vi "Increment Reported Error.vi"(4 "Newly Reported Error":T1, 5 "Module Data in":T3) -> (0 "Index of the newly reported error in the OSI data structure":i32, 1 "No. of times the error was handled in the last second":u32, 2 "Module Data out (OSI data updated)":T3)   [LabVIEW 2023, in "Error Manager.lvlib"]
doc: "Blank VI with error handling."
uses:
  Error Manager.lvlib
  Module Data (cluster).ctl
  Handled Error (cluster).ctl
  Read-Unread Status (enum).ctl
  Display Order (enum).ctl
  Error in current one-second interval (cluster).ctl
  Reported Error (cluster).ctl
  Public API VIs/Pop-up New Error Dialogue Instruction (enum).ctl
panel:
  # "Input\nInputs to the VI"
  # "Development\nControls or indicators that are useful for development or testing, but which are not outputs of the VI."
  # "Output\nOutputs of the VI"
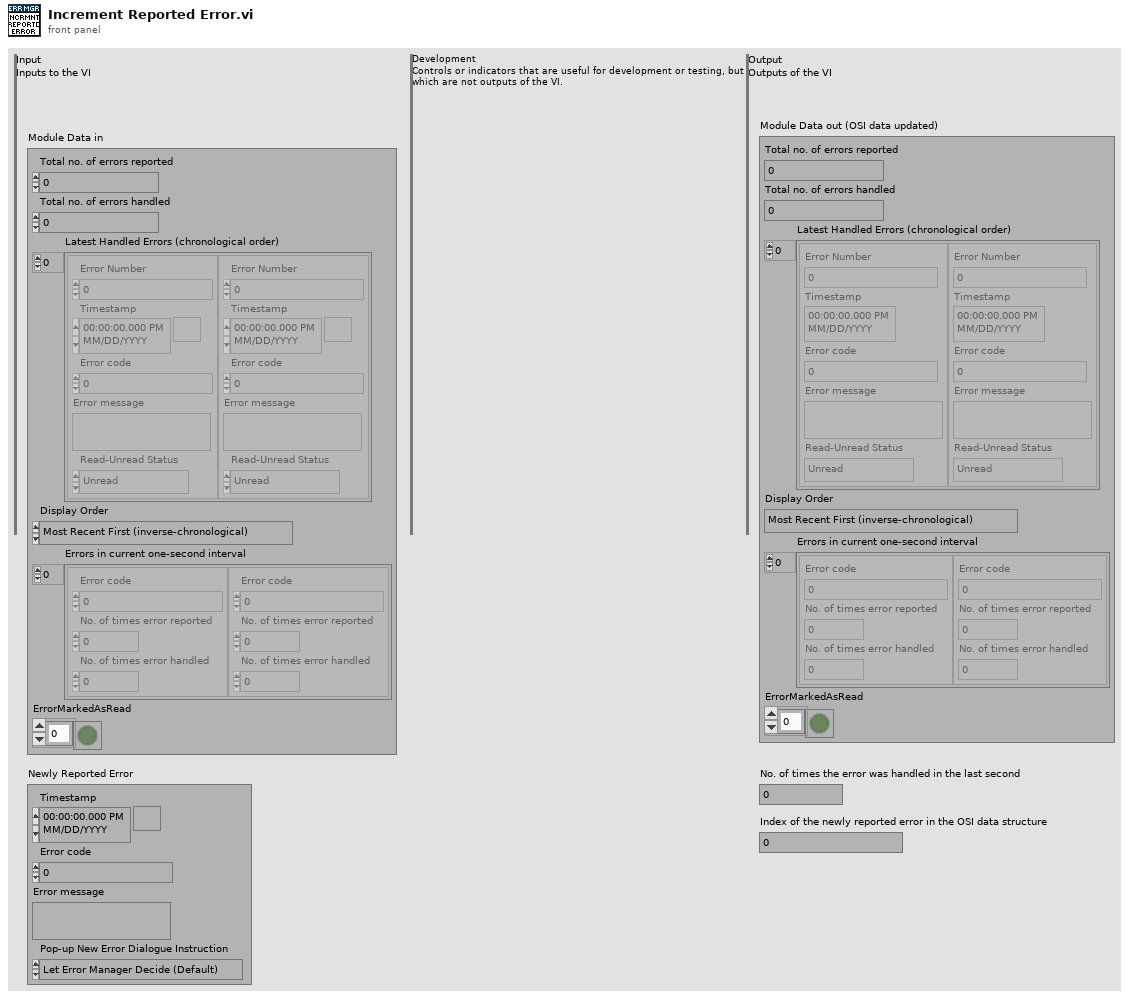
[diagram p1: front panel]
types:
  T1 = typedef "Error Manager.lvlib/Reported Error (cluster).ctl" = cluster{"Timestamp":timestamp, "Error code":i32, "Error message":string, "Pop-up New Error Dialogue Instruction":T2}
  T2 = typedef "Error Manager.lvlib/Pop-up New Error Dialogue Instruction (enum).ctl" = enum16{"Let Error Manager Decide (Default)", "Don't pop-up", "Pop-up"}
  T3 = typedef "Error Manager.lvlib/Module Data (cluster).ctl" = cluster{"Total no. of errors reported":i32, "Total no. of errors handled":i32, "Latest Handled Errors (chronological order)":T4[], "Display Order":T6, "Errors in current one-second interval":T7[], "ErrorMarkedAsRead":bool[]}
  T4 = typedef "Error Manager.lvlib/Handled Error (cluster).ctl" = cluster{"Error Number":i32, "Timestamp":timestamp, "Error code":i32, "Error message":string, "Read-Unread Status":T5}
  T5 = typedef "Error Manager.lvlib/Read-Unread Status (enum).ctl" = enum16{"Unread", "Read"}
  T6 = typedef "Error Manager.lvlib/Display Order (enum).ctl" = enum16{"Most Recent First (inverse-chronological)", "Oldest First (chronological)"}
  T7 = typedef "Error Manager.lvlib/Error in current one-second interval (cluster).ctl" = cluster{"Error code":i32, "No. of times error reported":u32, "No. of times error handled":u32}
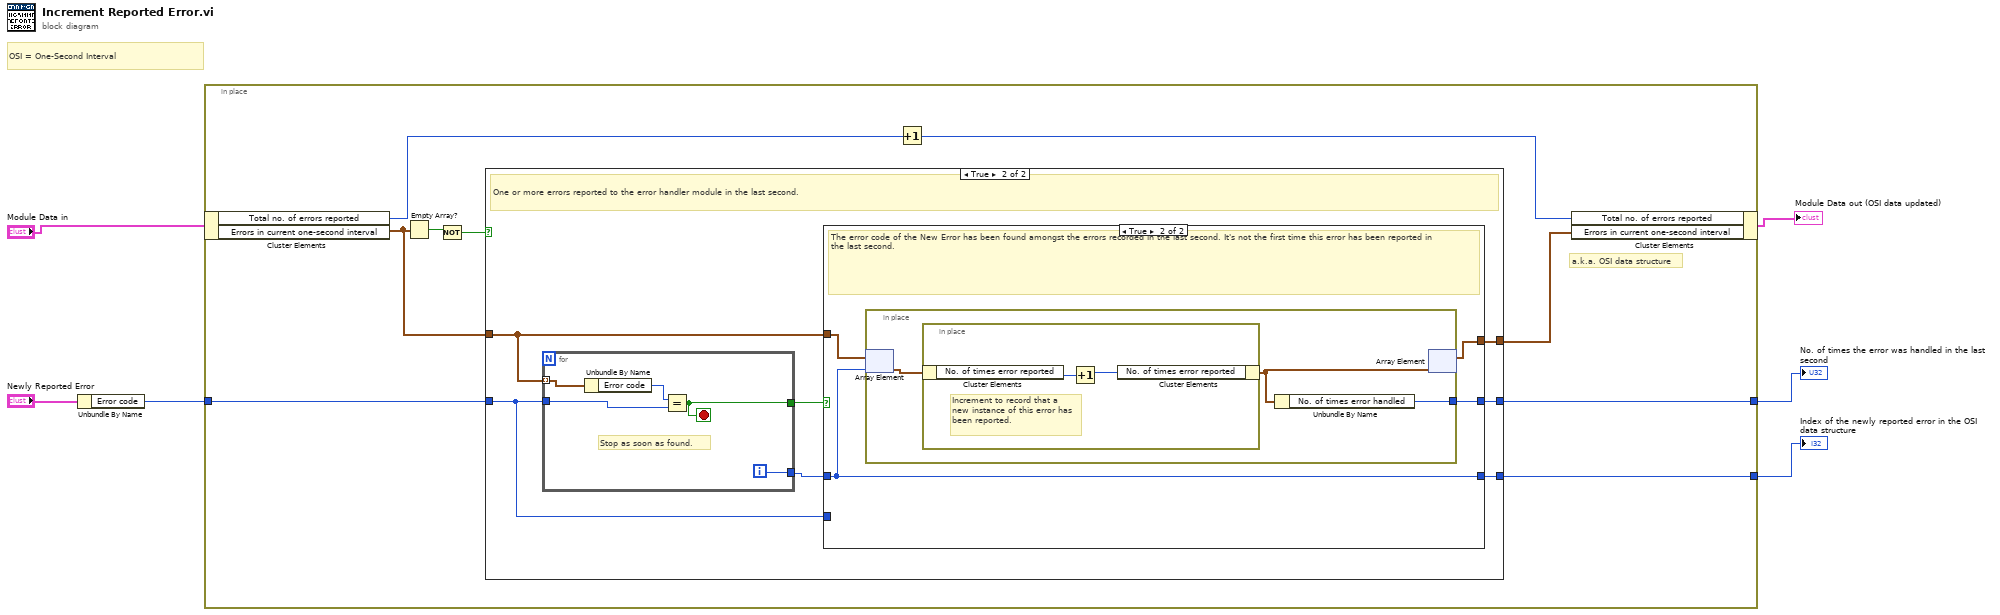
[diagram p0: block diagram]
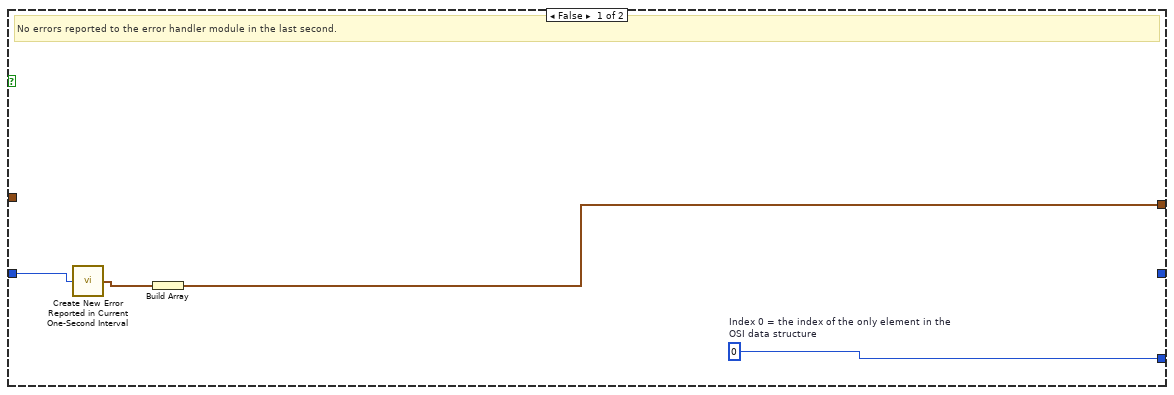
[diagram p2: hidden frame]
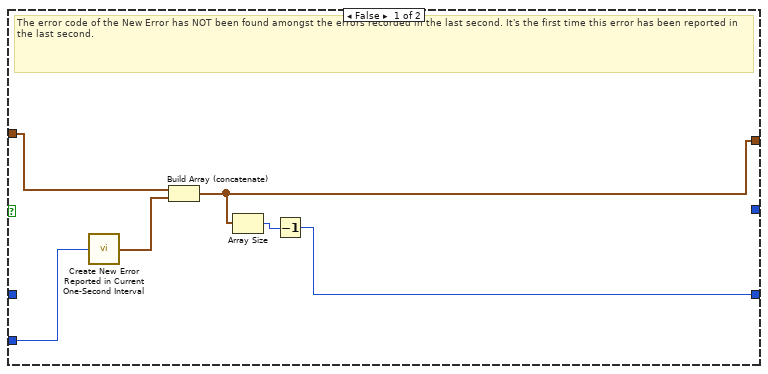
[diagram p3: hidden frame]
diagram:
  # "OSI = One-Second Interval"
  n1 = Unbundle By Name("Newly Reported Error") -> ("Error code"=w5:i32)
  n2 = in-place {
    in-place-border: w5 -> [w13]
    in-place-border: [w10] -> w2
    in-place-border: [w9] -> w1
    # "a.k.a. OSI data structure"
    n3 = in-place-cluster #1("Module Data in") -> ("Total no. of errors reported"=w8:i32, "Errors in current one-second interval"=w11:T7[])
    n4 = Empty Array?(array=w11) -> (empty?=w15:bool)
    n5 = Not(x=w15) -> (.not. x?=w14:bool)
    n6 = case shown="True" w14 {
      tunnel: w13 -> [w18 w21]
      tunnel: [w19 w22] -> w12
      tunnel: w11 -> [_ w23]
      tunnel: [w16 w24] -> w10
      tunnel: [_ w20] -> w9
      frame False {
        w16 = 0  # Index 0 = the index of the only element in the OSI data structure
        # "No errors reported to the error handler module in the last second."
        n7 = call "Create New Error Reported in Current One-Second Interval.vi"("Error code"=w18) -> ("Error in Current One-Second Interval"=w17:T7)
        n8 = Build Array(w17) -> (w19:T7[])
      }
      frame True {
        # "One or more errors reported to the error handler module in the last second."
        n9 = for {
          tunnel: w23 -> [w46] mode=indexing
          tunnel: w21 -> [w44]
          tunnel: [w43] -> w26
          tunnel: [w42] -> w25
          i -> [w42]
          stop <- w43 stop-if-true
          # "Stop as soon as found."
          n10 = Unbundle By Name(w46) -> ("Error code"=w45:i32)
          n11 = Equal?(x=w45, y=w44) -> (x = y?=w43:bool)
        }
        n12 = case shown="True" w26 {
          tunnel: w25 -> [_ w35]
          tunnel: [w27 w35] -> w24
          tunnel: w23 -> [w32 w36]
          tunnel: [w29 w34] -> w22
          tunnel: w21 -> [w30 _]
          tunnel: [_ w33] -> w20
          frame False {
            # "The error code of the New Error has NOT been found amongst the errors recorded in the last second. It's the first time this error has been reported in the last second."
            n13 = call "Create New Error Reported in Current One-Second Interval.vi"("Error code"=w30) -> ("Error in Current One-Second Interval"=w31:T7)
            n14 = Build Array (concatenate)(w32, w31) -> (w29:T7[])
            n15 = Array Size(array=w29) -> (size(s)=w28:i32)
            n16 = Decrement(x=w28) -> (x-1=w27:i32)
          }
          frame True {
            # "The error code of the New Error has been found amongst the errors recorded in the last second. It's not the first time this error has been reported in the last second."
            n17 = in-place {
              in-place-border: [w37] -> w33
              n18 = in-place-array #2(w36, w35) -> (w39:T7)
              n19 = in-place {
                # "Increment to record that a new instance of this error has been reported."
                n20 = in-place-cluster #3(w39) -> ("No. of times error reported"=w41:u32)
                n21 = Increment(x=w41) -> (x+1=w40:u32)
                n22 = in-place-cluster #3("No. of times error reported"=w40) -> (w38:T7)
              }
              n23 = Unbundle By Name(w38) -> ("No. of times error handled"=w37:u32)
              n24 = in-place-array #2(w38) -> (w34:T7[])  [unwired: 1 out]
            }
          }
        }
      }
    }
    n25 = Increment(x=w8) -> (x+1=w7:i32)
    n26 = in-place-cluster #1("Total no. of errors reported"=w7, "Errors in current one-second interval"=w12) -> (→"Module Data out (OSI data updated)":T3)
  }
  "No. of times the error was handled in the last second" <- w1
  "Index of the newly reported error in the OSI data structure" <- w2
